vi "Search Optimization.vi"() -> ()   [LabVIEW 2020, in "NI_VIAnCFGDataStructure.lvlib" / "Tree.lvclass"]
uses:
  <vilib>/addons/analyzer/VIAnCFGDataStructure/Tree Manager/Tree.lvclass
panel:
  out "Results Valid":bool=TRUE
  out "Impr. minus Optimization Time":dbl=0.0933169201889541 format="%#.1p"
  out "Speed Improvement":dbl=0.09704901871737093 format="%#.1p"
  out "Creation Time":dbl=0.002733134519075975 format="%#.1p"
  out "UI Drawing Time":dbl=0.034517327236244455 format="%#.1p"
  out "Unoptimized Search":dbl=0.09730149249662645 format="%#.1p"
  out "Optimization Time":dbl=0.0037320985284168273 format="%#.1p"
  out "Optimized Search":dbl=0.0002524737792555243 format="%#.1p"
  out "# Search Paths":i32=125
  in  "Tree":string(tree)="Root"
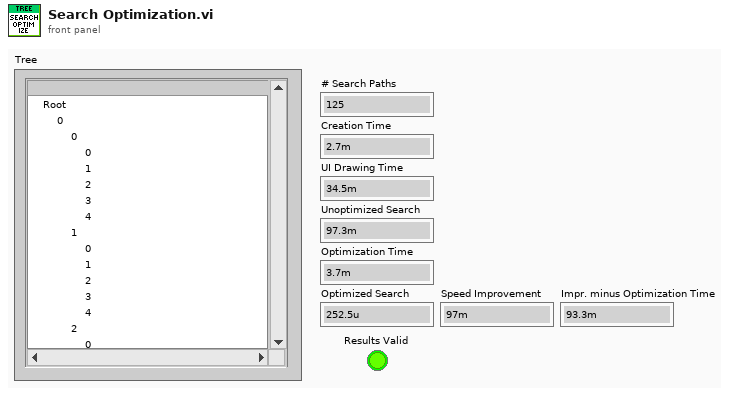
[diagram p1: front panel]
types:
  T1 = typedef "NI_VIAnCFGDataStructure.lvlib/Tree.lvclass/Session Handle.ctl" = refnum<data-value>
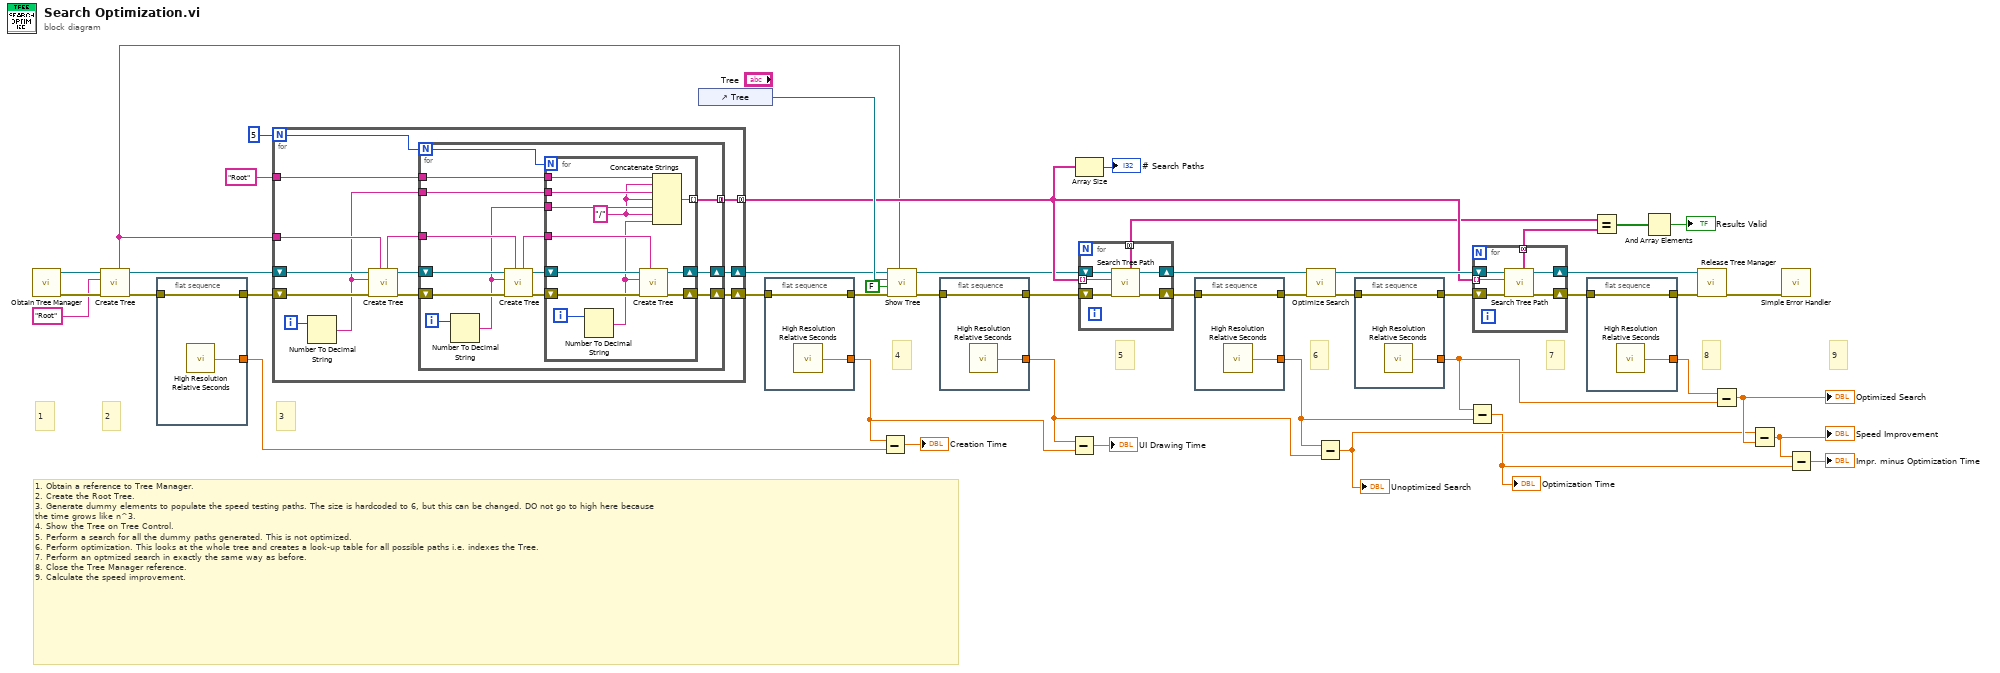
[diagram p0: block diagram]
diagram:
  # "1. Obtain a reference to Tree Manager.\n2. Create the Root Tree.\n3. Generate dummy elements to populate the speed testing paths. The size is hardcoded to 6, but this can be changed. DO not go to high here because\nthe time grows like n^3.\n4. Show the Tree on Tree Control.\n5. Perform a search for all the dummy paths generated. This is not optimized.\n6. Perform optimization. This looks at the whole tree and creates a look-up table for all possible paths i.e. indexes the Tree.\n7. Perform an optmized search in exactly the same way as before.\n8. Close the Tree Manager reference.\n9. Calculate the speed improvement."
  # "9"
  # "8"
  # "7"
  # "6"
  # "5"
  # "4"
  # "3"
  # "2"
  # "1"
  n1 = call <vilib>:"Obtain Tree Manager.vi"() -> ("Error Out"=w45:errorcluster, "Tree"=w46:T1)  [unwired: 10 in]
  n2 = call <vilib>:"Create Tree.vi"("Error In"=w45, "Name"="Root", "Tree Manager"=w46) -> ("Error Out"=w39:errorcluster, "Tree Manager"=w42:T1, "Unique ID"=w6:string)  [unwired: 6 in]
  n3 = flat-sequence {
    tunnel: [w48] -> w40
    tunnel: w39 -> [w48]
    tunnel: [w47] -> w21
    frame #0 {
      n4 = call <vilib>:"High Resolution Relative Seconds.vi"() -> ("relative seconds"=w47:dbl)
    }
  }
  n5 = for {
    N: 5 -> [w52]
    shift-right: [w54] -> w19
    shift-left: w42 -> [w61]
    shift-right: [w53] -> w17
    shift-left: w40 -> [w60]
    tunnel: w6 -> [w59]
    tunnel: "Root" ("Name") -> [w51]
    tunnel: [w49] -> w15 mode=concatenating
    i -> [w58]
    n6 = Number To Decimal String(number=w58) -> (decimal integer string=w50:string)  [unwired: 1 in]
    n7 = call <vilib>:"Create Tree.vi"("Parent ID (empty)"=w59, "Error In"=w60, "Name"=w50, "Tree Manager"=w61) -> ("Error Out"=w55:errorcluster, "Tree Manager"=w57:T1, "Unique ID"=w56:string)  [unwired: 5 in]
    n8 = for {
      N: w52 -> [w68]
      shift-right: [w67] -> w54
      shift-left: w57 -> [w75]
      tunnel: w56 -> [w74]
      shift-right: [w66] -> w53
      shift-left: w55 -> [w72]
      tunnel: w51 -> [w65]
      tunnel: w50 -> [w64]
      tunnel: [w62] -> w49 mode=concatenating
      i -> [w73]
      n9 = Number To Decimal String(number=w73) -> (decimal integer string=w63:string)  [unwired: 1 in]
      n10 = call <vilib>:"Create Tree.vi"("Parent ID (empty)"=w74, "Error In"=w72, "Name"=w63, "Tree Manager"=w75) -> ("Error Out"=w69:errorcluster, "Tree Manager"=w71:T1, "Unique ID"=w70:string)  [unwired: 5 in]
      n11 = for {
        N: w68 -> [_]
        tunnel: w70 -> [w85]
        shift-right: [w82] -> w66
        shift-left: w69 -> [w84]
        shift-right: [w83] -> w67
        shift-left: w71 -> [w86]
        tunnel: w65 -> [w81]
        tunnel: w64 -> [w80]
        tunnel: w63 -> [w79]
        tunnel: [w76] -> w62 mode=indexing
        i -> [w87]
        w78 = "/" ("string")
        n12 = Number To Decimal String(number=w87) -> (decimal integer string=w77:string)  [unwired: 1 in]
        n13 = call <vilib>:"Create Tree.vi"("Parent ID (empty)"=w85, "Error In"=w84, "Name"=w77, "Tree Manager"=w86) -> ("Error Out"=w82:errorcluster, "Tree Manager"=w83:T1)  [unwired: 5 in, 1 out]
        n14 = Concatenate Strings(w81, w78, w80, w78, w79, w78, w77) -> (w76:string)
      }
    }
  }
  n15 = control-ref of="Tree"() -> (w41:refnum<vi>)
  n16 = flat-sequence {
    tunnel: [w89] -> w38
    tunnel: w17 -> [w89]
    tunnel: [w88] -> w8
    frame #0 {
      n17 = call <vilib>:"High Resolution Relative Seconds.vi"() -> ("relative seconds"=w88:dbl)
    }
  }
  n18 = Subtract(x=w8, y=w21) -> (x-y=→"Creation Time":dbl)
  n19 = call <vilib>:"Show Tree.vi"("Root ID"=w6, "Error In"=w38, "Show IDs (False)"=FALSE ("Show IDs (True)"), "Tree Ref"=w41, "Tree"=w19) -> ("Error Out"=w37:errorcluster, "Tree"=w7:T1)  [unwired: 5 in]
  n20 = flat-sequence {
    tunnel: [w91] -> w36
    tunnel: w37 -> [w91]
    tunnel: [w90] -> w18
    frame #0 {
      n21 = call <vilib>:"High Resolution Relative Seconds.vi"() -> ("relative seconds"=w90:dbl)
    }
  }
  n22 = Subtract(x=w18, y=w8) -> (x-y=→"UI Drawing Time":dbl)
  n23 = Array Size(array=w15) -> (size(s)=→"# Search Paths":i32)
  n24 = for {
    shift-right: [w94] -> w32
    shift-left: w7 -> [w97]
    shift-right: [w95] -> w35
    shift-left: w36 -> [w96]
    tunnel: w15 -> [w93] mode=indexing
    tunnel: [w92] -> w3 mode=concatenating
    n25 = call <vilib>:"Search Tree Path.vi"("Error In"=w96, "Tree Path"=w93, "Tree Manager"=w97) -> ("Error Out"=w95:errorcluster, "Tree Manager"=w94:T1, "Tree IDs"=w92:string[])  [unwired: 6 in]
  }
  n26 = flat-sequence {
    tunnel: [w99] -> w33
    tunnel: w35 -> [w99]
    tunnel: [w98] -> w23
    frame #0 {
      n27 = call <vilib>:"High Resolution Relative Seconds.vi"() -> ("relative seconds"=w98:dbl)
    }
  }
  n28 = call <vilib>:"Optimize Search.vi"("Error In"=w33, "Tree Manager"=w32) -> ("Error Out"=w31:errorcluster, "Tree Manager"=w29:T1)  [unwired: 8 in]
  n29 = Subtract(x=w23, y=w18) -> (x-y=w13:dbl)
  "Unoptimized Search" <- w13
  n30 = flat-sequence {
    tunnel: [w101] -> w30
    tunnel: w31 -> [w101]
    tunnel: [w100] -> w24
    frame #0 {
      n31 = call <vilib>:"High Resolution Relative Seconds.vi"() -> ("relative seconds"=w100:dbl)
    }
  }
  n32 = Subtract(x=w24, y=w23) -> (x-y=w9:dbl)
  "Optimization Time" <- w9
  n33 = for {
    shift-right: [w104] -> w27
    shift-left: w29 -> [w107]
    shift-right: [w105] -> w28
    shift-left: w30 -> [w106]
    tunnel: w15 -> [w103] mode=indexing
    tunnel: [w102] -> w2 mode=concatenating
    n34 = call <vilib>:"Search Tree Path.vi"("Error In"=w106, "Tree Path"=w103, "Tree Manager"=w107) -> ("Error Out"=w105:errorcluster, "Tree Manager"=w104:T1, "Tree IDs"=w102:string[])  [unwired: 6 in]
  }
  n35 = flat-sequence {
    tunnel: [w109] -> w26
    tunnel: w28 -> [w109]
    tunnel: [w108] -> w25
    frame #0 {
      n36 = call <vilib>:"High Resolution Relative Seconds.vi"() -> ("relative seconds"=w108:dbl)
    }
  }
  n37 = Equal?(x=w3, y=w2) -> (x = y?=w5:bool[])
  n38 = And Array Elements(Boolean array=w5) -> (logical AND=→"Results Valid":bool)
  n39 = call <vilib>:"Release Tree Manager.vi"("Error In"=w26, "Tree"=w27) -> ("Error Out"=w1:errorcluster)  [unwired: 9 in]
  n40 = Subtract(x=w25, y=w24) -> (x-y=w14:dbl)
  "Optimized Search" <- w14
  n41 = Subtract(x=w13, y=w14) -> (x-y=w12:dbl)
  "Speed Improvement" <- w12
  n42 = call <vilib>:"Simple Error Handler.vi"("error in (no error)"=w1) -> ()  [unwired: 4 in, 5 out]
  n43 = Subtract(x=w12, y=w9) -> (x-y=→"Impr. minus Optimization Time":dbl)
